vi "KT.vi"(3 "Channel input":dbl=2.0, 4 "TaskIn":string="SET START", 6 "error in (no error)":errorcluster) -> (0 "CommandOut":string, 2 "error out":errorcluster)   [LabVIEW 2018]
doc: "Use this template to build a VI to use as a subVI."
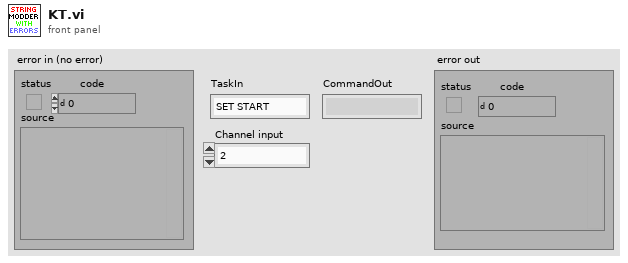
[diagram p1: front panel]
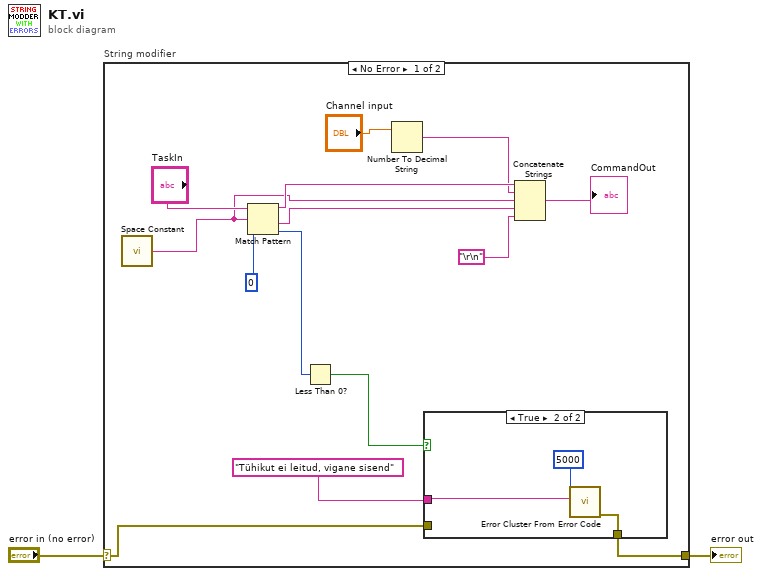
[diagram p0: block diagram]
diagram:
  n1 = case "String modifier" shown="No Error" "error in (no error)" {
    selector: "error in (no error)" -> [w13 w20]
    tunnel: [w14 w20] -> w1
    frame No Error {
      n2 = call <vilib>:"Space Constant.vi"() -> ("String"=w8:string)
      n3 = Match Pattern(string="TaskIn", regular expression=w8, offset (0)=0) -> (before substring=w9:string, after substring=w7:string, offset past match=w12:i32)  [unwired: 1 out]
      n4 = Less Than 0?(x=w12) -> (x < 0?=w11:bool)
      n5 = Number To Decimal String(number="Channel input") -> (decimal integer string=w4:string)  [unwired: 1 in]
      n6 = case shown="True" w11 {
        tunnel: [_ w19] -> w14
        tunnel: w13 -> [_ _]
        tunnel: "Tühikut ei leitud, vigane sisend" ("Error message") -> [_ w17]
        frame False {
        }
        frame True {
          n7 = call <vilib>:"Error Cluster From Error Code.vi"("error message (\"\")"=w17, "error code (0)"=5000) -> ("error out"=w19:errorcluster)  [unwired: 7 in]
        }
      }
      n8 = Concatenate Strings(w9, w4, w8, w7, "\r\n") -> (→"CommandOut":string)
    }
    frame Error {
    }
  }
  "error out" <- w1
